vi "Reload Plot Property.vi"(6 "Sub VI":refnum<vi>, 8 "error in (no error)":errorcluster, 11 "Plot Property Array In":T1) -> (0 "error out":errorcluster, 3 "Plot Property Array Out":T1)   [LabVIEW 2020, in "XY Plot Matrix.lvclass"]
uses:
  <vilib>/Math Plots/2D Math Plots/XY Plot Matrix/XY Plot Matrix/XY Plot Matrix.lvclass
  <vilib>/Math Plots/2D Math Plots/XY Plot Matrix/XY Plot Matrix/Typedef/Plotmatrix Property Array.ctl
  <vilib>/Math Plots/2D Math Plots/XY Plot Matrix/XY Plot Matrix/Typedef/Plotmatrix Property.ctl
  <vilib>/Math Plots/2D Math Plots/2D Plot/2D Plot/Typedef/Plot Property Array.ctl
  <vilib>/Math Plots/2D Math Plots/2D Plot/2D Plot/Typedef/Plot Property.ctl
  <vilib>/Math Plots/2D Math Plots/2D Plot/2D Plot/2D Plot.lvclass
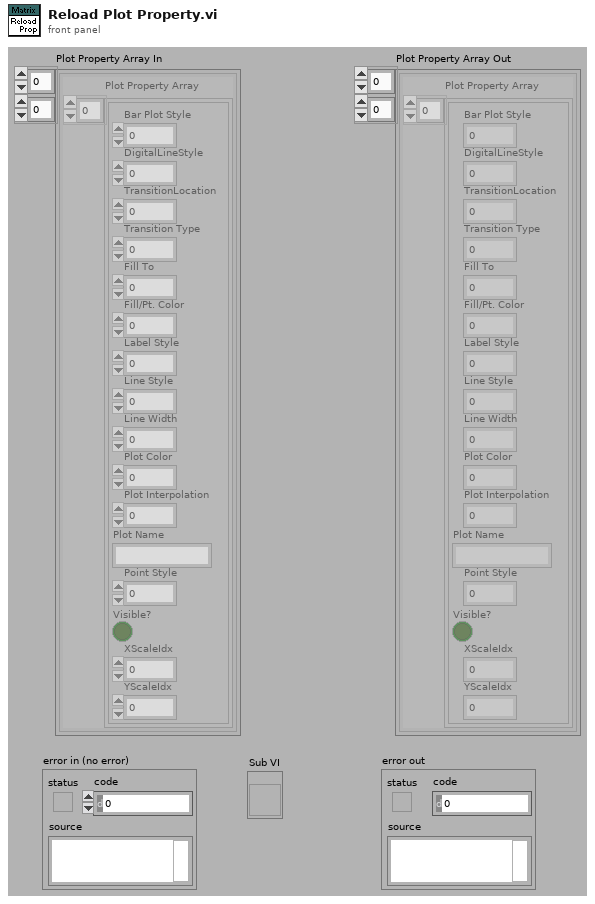
[diagram p1: front panel]
types:
  T1 = typedef "XY Plot Matrix.lvclass/Plotmatrix Property Array.ctl" = T2[][]
  T2 = typedef "XY Plot Matrix.lvclass/Plotmatrix Property.ctl" = cluster{"Plot Property Array":T3}
  T3 = typedef "2D Plot.lvclass/Plot Property Array.ctl" = T4[]
  T4 = typedef "2D Plot.lvclass/Plot Property.ctl" = cluster{"Bar Plot Style":u8, "DigitalLineStyle":u8, "TransitionLocation":u8, "Transition Type":u8, "Fill To":i16, "Fill/Pt. Color":u32, "Label Style":u8, "Line Style":u8, "Line Width":u8, "Plot Color":u32, "Plot Interpolation":u8, "Plot Name":string, "Point Style":u8, "Visible?":bool, "XScaleIdx":u32, "YScaleIdx":u32}
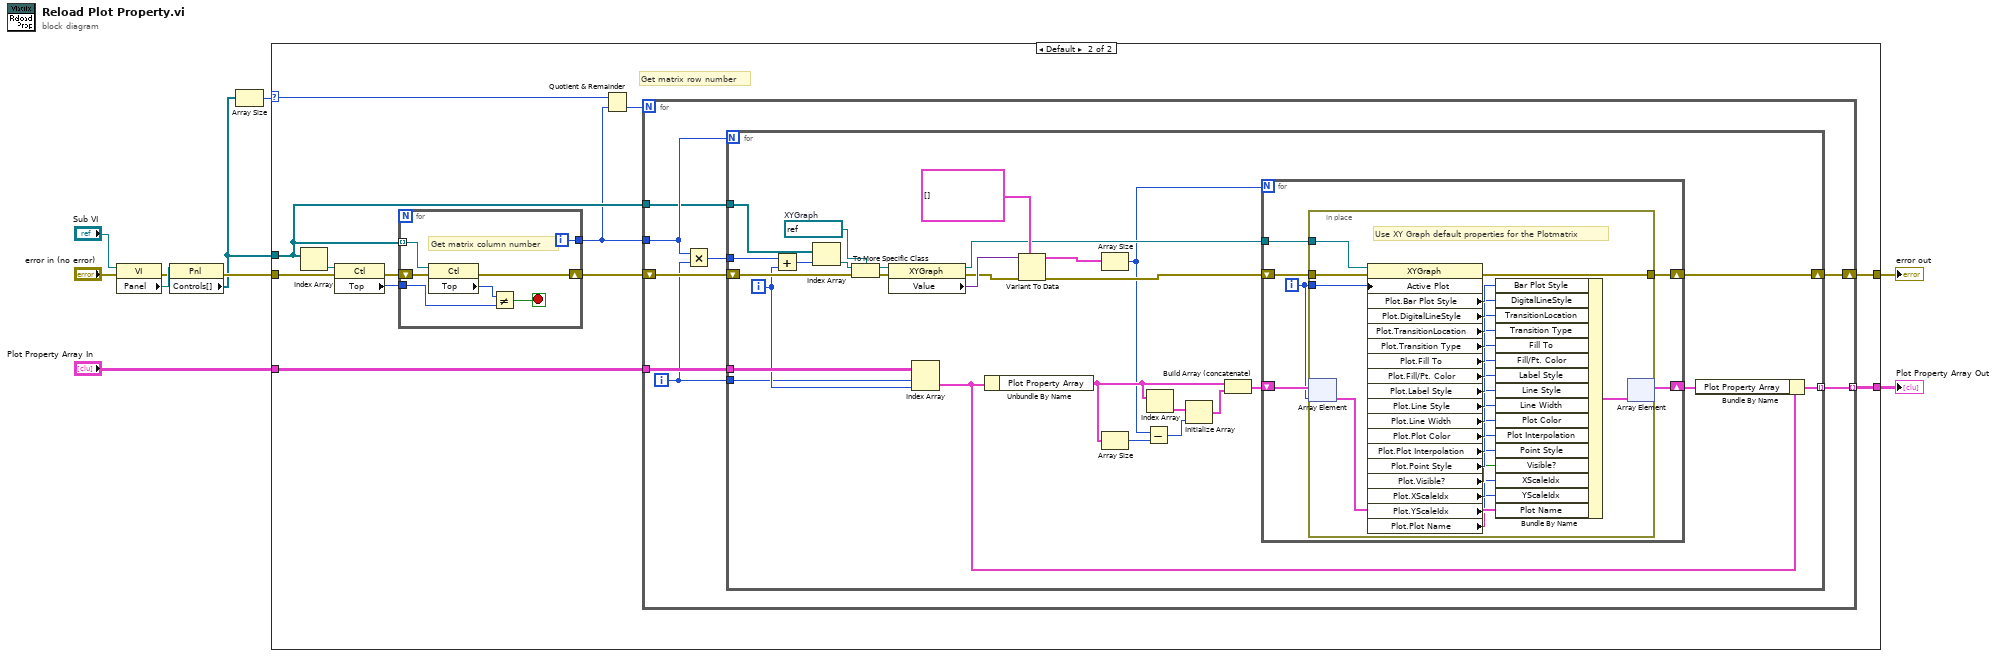
[diagram p0: block diagram]
diagram:
  n1 = property class="VI"(reference="Sub VI", error in="error in (no error)") -> (error out=w7:errorcluster, "Panel"=w9:refnum<vi>)  [unwired: 1 out]
  n2 = property class="Pnl"(reference=w9, error in=w7) -> (error out=w5:errorcluster, "Controls[]"=w2:refnum<vi>[])  [unwired: 1 out]
  n3 = Array Size(array=w2) -> (size(s)=w1:i32)
  n4 = case shown="Default" w1 {
    selector: w1 -> [_ w13]
    tunnel: [w11 w24] -> w10
    tunnel: w5 -> [w11 w22]
    tunnel: "Plot Property Array In" -> [w12 w20]
    tunnel: [w12 w18] -> w3
    tunnel: w2 -> [_ w17]
    frame 0 {
    }
    frame Default {
      # "Get matrix row number"
      n5 = Index Array(array=w17) -> (element=w23:refnum<vi>)  [unwired: 1 in]
      n6 = property class="Ctl"(reference=w23, error in=w22) -> (error out=w16:errorcluster, "Top"=w21:i32)  [unwired: 1 out]
      n7 = for {
        tunnel: w17 -> [w95] mode=indexing
        tunnel: w21 -> [w93]
        tunnel: [w91] -> w14
        shift-right: [w89] -> w15
        shift-left: w16 -> [w90]
        i -> [w91]
        stop <- w92 stop-if-true
        # "Get matrix column number"
        n8 = property class="Ctl"(reference=w95, error in=w90) -> (error out=w89:errorcluster, "Top"=w94:i32)  [unwired: 1 out]
        n9 = Not Equal?(x=w94, y=w93) -> (x != y?=w92:bool)
      }
      n10 = Quotient & Remainder(x=w13, y=w14) -> (floor(x/y)=w19:i32)  [unwired: 1 out]
      n11 = for {
        N: w19 -> [_]
        tunnel: w17 -> [w28]
        tunnel: w20 -> [w31]
        tunnel: w14 -> [w29]
        tunnel: [w30] -> w18 mode=indexing
        shift-right: [w32] -> w24
        shift-left: w15 -> [w26]
        i -> [w25]
        n12 = Multiply(x=w29, y=w25) -> (x*y=w27:i32)
        n13 = for {
          N: w29 -> [_]
          tunnel: w31 -> [w42]
          tunnel: [w47] -> w30 mode=indexing
          tunnel: w28 -> [w46]
          tunnel: w27 -> [w39]
          shift-right: [w60] -> w32
          shift-left: w26 -> [w43]
          tunnel: w25 -> [w38]
          i -> [w40]
          w58 = refnum<vi> refnum  # XYGraph
          n14 = Add(x=w39, y=w40) -> (x+y=w45:i32)
          n15 = Index Array(array=w46, index=w45) -> (element=w44:refnum<vi>)
          n16 = To More Specific Class(target class=w58, reference=w44, error in=w43) -> (specific class reference=w54:refnum<vi>, error out=w50:errorcluster)
          n17 = property class="XYGraph"(reference=w54, error in=w50) -> (reference out=w52:refnum<vi>, error out=w55:errorcluster, "Value"=w57:variant)
          n18 = Index Array(array=w42, index (row)=w38, index (col)=w40) -> (element=w41:T2)
          n19 = Unbundle By Name(w41) -> ("Plot Property Array"=w49:T3)
          n20 = Variant To Data(error in=w55, type=cluster{"X":dbl[], "Y":dbl[]}[] [] ("appended array"), Variant=w57) -> (data=w53:cluster{"X":dbl[], "Y":dbl[]}[], error out=w51:errorcluster)
          n21 = Array Size(array=w53) -> (size(s)=w33:i32)
          n22 = Array Size(array=w49) -> (size(s)=w59:i32)
          n23 = Subtract(x=w33, y=w59) -> (x-y=w34:i32)
          n24 = Index Array(array=w49) -> (element=w37:T4)  [unwired: 1 in]
          n25 = Initialize Array(w37, w34) -> (w36:T4[])
          n26 = Build Array (concatenate)(w49, w36) -> (w35:T3)
          n27 = for {
            N: w33 -> [_]
            tunnel: w52 -> [w62]
            shift-right: [w65] -> w48
            shift-left: w35 -> [w66]
            shift-right: [w63] -> w60
            shift-left: w51 -> [w64]
            i -> [w61]
            n28 = in-place {
              in-place-border: w62 -> [w86]
              in-place-border: w61 -> [w85]
              in-place-border: w64 -> [w69]
              in-place-border: [w68] -> w63
              # "Use XY Graph default properties for the Plotmatrix"
              n29 = in-place-array #1(w66, w61) -> (w88:T4)
              n30 = property class="XYGraph"(reference=w86, error in=w69, "Active Plot"=w85) -> (error out=w68:errorcluster, "Plot.Bar Plot Style"=w84:u8, "Plot.DigitalLineStyle"=w83:u8, "Plot.TransitionLocation"=w82:u8, "Plot.Transition Type"=w81:u8, "Plot.Fill To"=w80:i16, "Plot.Fill/Pt. Color"=w79:u32, "Plot.Label Style"=w78:u8, "Plot.Line Style"=w77:u8, "Plot.Line Width"=w76:u8, "Plot.Plot Color"=w75:u32, "Plot.Plot Interpolation"=w74:u8, "Plot.Point Style"=w73:u8, "Plot.Visible?"=w72:bool, "Plot.XScaleIdx"=w71:u32, "Plot.YScaleIdx"=w70:u32, "Plot.Plot Name"=w67:string)  [unwired: 1 out]
              n31 = Bundle By Name(cluster=w88, "Bar Plot Style"=w84, "DigitalLineStyle"=w83, "TransitionLocation"=w82, "Transition Type"=w81, "Fill To"=w80, "Fill/Pt. Color"=w79, "Label Style"=w78, "Line Style"=w77, "Line Width"=w76, "Plot Color"=w75, "Plot Interpolation"=w74, "Point Style"=w73, "Visible?"=w72, "XScaleIdx"=w71, "YScaleIdx"=w70, "Plot Name"=w67) -> (w87:T4)
              n32 = in-place-array #1(w87) -> (w65:T3)  [unwired: 1 out]
            }
          }
          n33 = Bundle By Name(cluster=w41, "Plot Property Array"=w48) -> (w47:T2)
        }
      }
    }
  }
  "Plot Property Array Out" <- w3
  "error out" <- w10
